vi "Command Editor Dialog.vi"(7 "Name(\"\" to use uuid)":string="Event CSM Tiny", 8 "Error in":errorcluster caption="Error in (no error)", 11 "Command":string="UI: Front Panel State >> Open -@ abc") -> (0 "Error out":errorcluster, 3 "Command out":string)   [LabVIEW 2017]
uses:
  _Polymophic/Build Message with Arguments(Auto Check).vi
  _Support/Common/Trim Single line Text.vi
  AdvanceAPI/CSM - Break Down Multiple States String.vi
  AdvanceAPI/CSM - Compact Multiple States.vi
  AdvanceAPI/CSM - Keywords.vi
  _Support/CSMQ/_CSMOFGV.vi
  _Support/Message/Parse State with Arguments String.vi
  Communicable State Machine.lvlib
  _csmHelper/API with lvcsm Support/CSM-Helper API with lvcsm Support.lvlib
panel:
  in  "State":string(combo)
  in  "Argument":string(combo)
  in  "symbol":string(combo)
  in  "Target":string(combo)
  in  "Comments":string
  in  "CSM VI Def":string(combo)
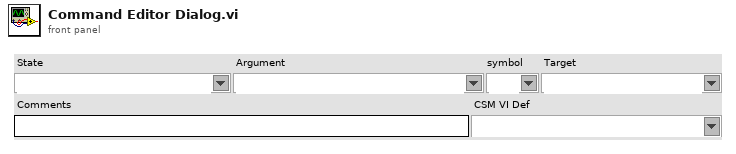
[diagram p1: front panel]
types:
  T1 = enum32{"Invalid", "Standard", "Closed", "Hidden", "Minimized", "Maximized"}
  T2 = enum32{"invalid app kind", "Development System", "Run Time System", "Student Edition", "Embedded LabVIEW", "Evaluation", "Custom"}
  T3 = typedef "Communicable State Machine.lvlib/_CSM_Response Source Message.ctl" = cluster{"‘State":string, "’Arguments":string, "’Error":errorcluster}
  T4 = cluster{"Current VI Reference":refnum<vi>, "Close Panel on Exit?":bool}
  T5 = cluster{"Core":cluster{"Current VI Reference":refnum<vi>, "Close Panel on Exit?":bool}, "Command":string}
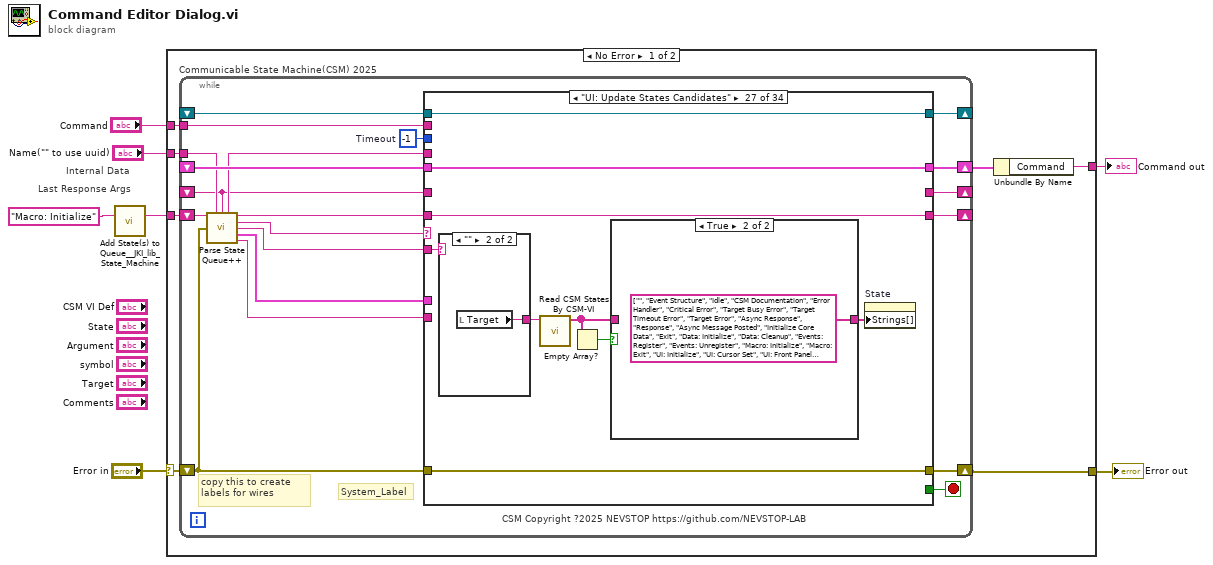
[diagram p0: block diagram]
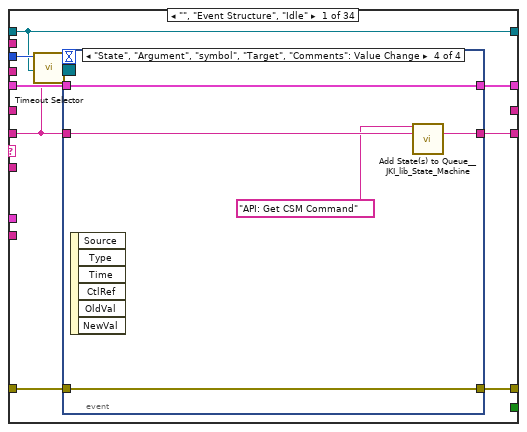
[diagram p2: hidden frame]
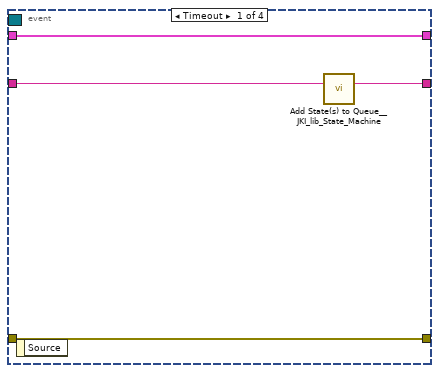
[diagram p3: hidden frame]
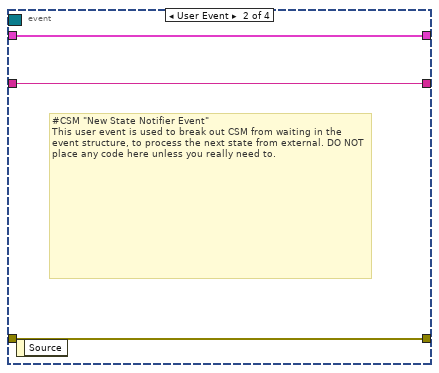
[diagram p4: hidden frame]
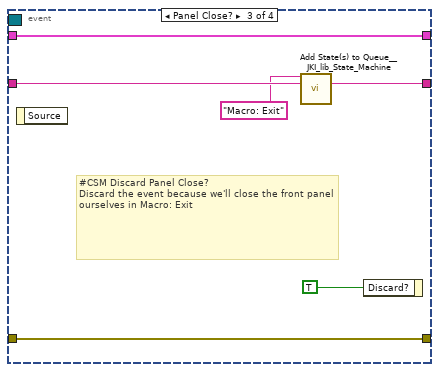
[diagram p5: hidden frame]
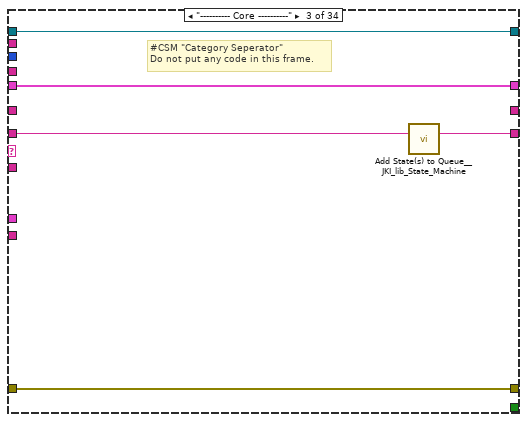
[diagram p7: hidden frame]
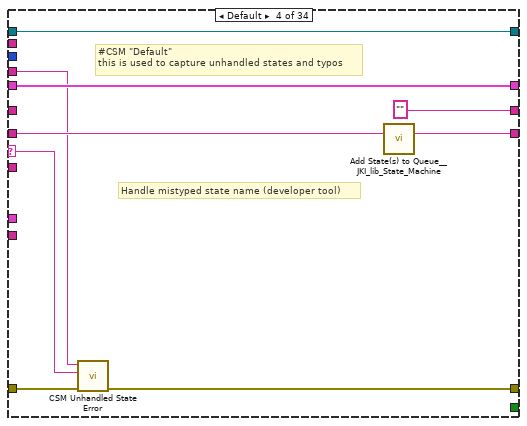
[diagram p8: hidden frame]
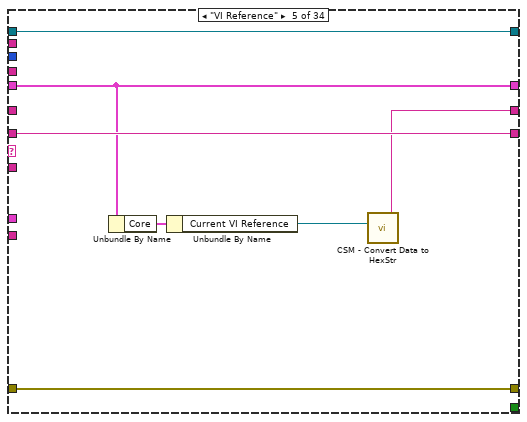
[diagram p9: hidden frame]
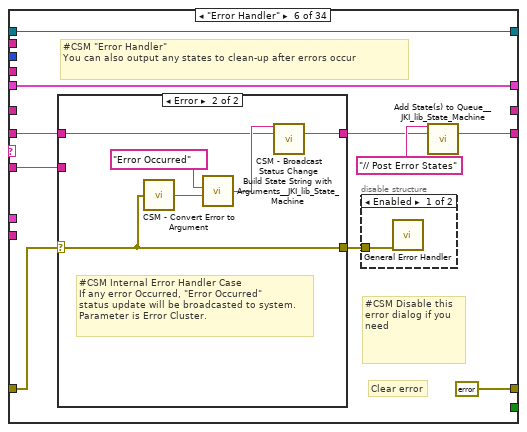
[diagram p10: hidden frame]
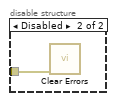
[diagram p11: hidden frame]
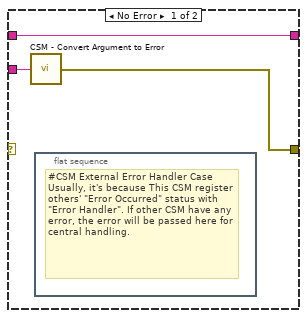
[diagram p12: hidden frame]
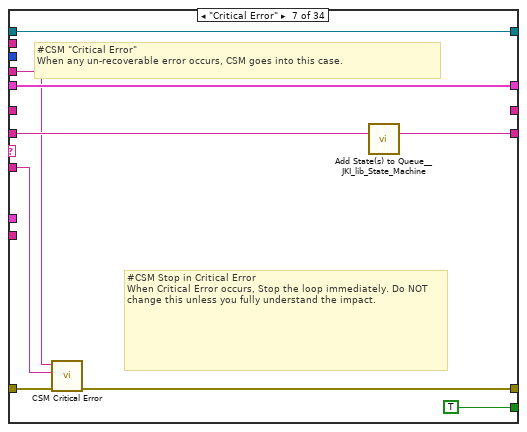
[diagram p13: hidden frame]
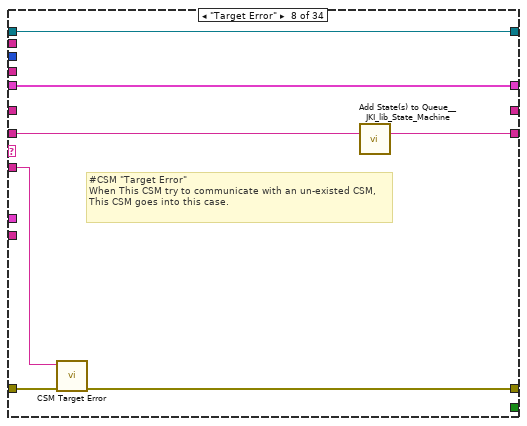
[diagram p14: hidden frame]
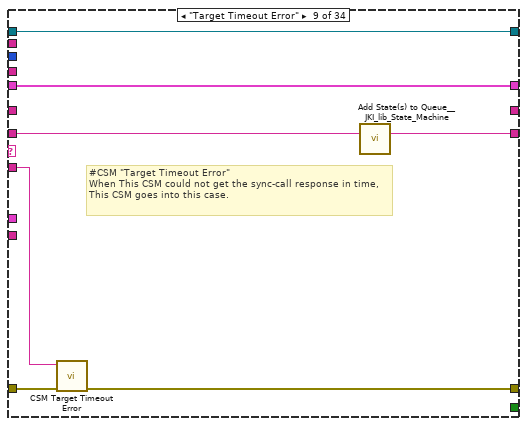
[diagram p15: hidden frame]
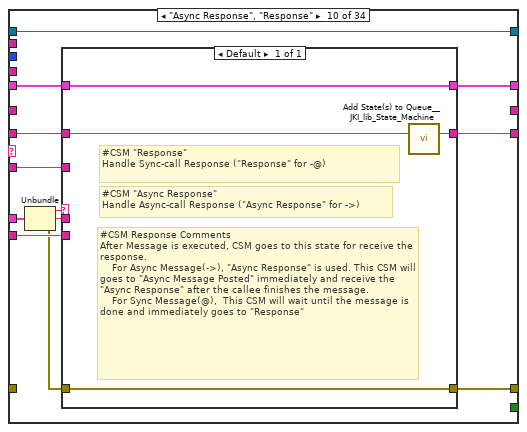
[diagram p16: hidden frame]
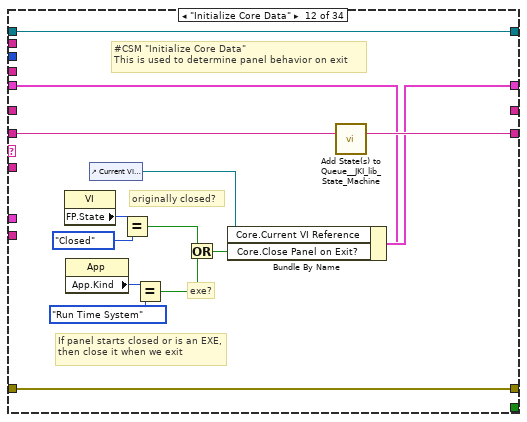
[diagram p18: hidden frame]
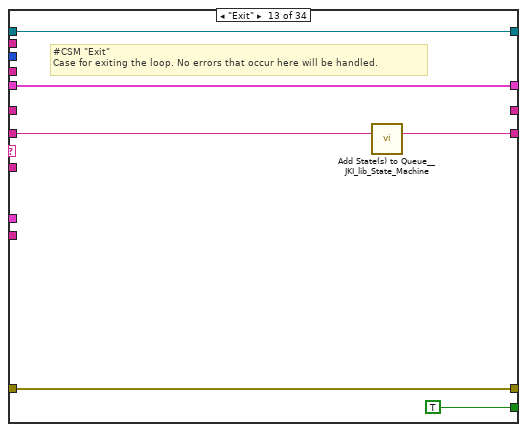
[diagram p19: hidden frame]
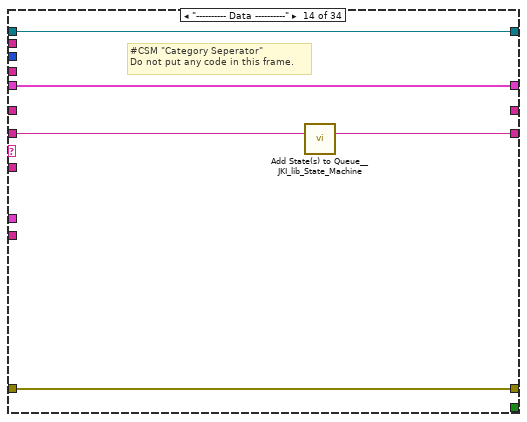
[diagram p20: hidden frame]
diagram:
  # "Last Response Args"
  # "Internal Data"
  n1 = call <vilib>:"Add State(s) to Queue__JKI_lib_State_Machine.vi"("State(s) in (\"\")"="Macro: Initialize" ("Init State(\"Macro: Initialize\")")) -> ("States Out"=w7:string)  [unwired: 14 in]
  n2 = case shown="No Error" "Error in" {
    selector: "Error in" -> [w11 w405]
    tunnel: w7 -> [w14 _]
    tunnel: "Name(\"\" to use uuid)" -> [w13 _]
    tunnel: [w12 w405] -> w4
    tunnel: [w9 w404] -> w2
    tunnel: "Command" -> [w8 w404]
    frame No Error {
      n3 = while "Communicable State Machine(CSM) 2025" {
        shift-right: [w29] -> w10
        shift-left: _ -> [w28]
        shift-right: [w32] -> w12
        shift-left: w11 -> [w26]
        shift-right: [w31] -> _
        shift-left: w14 -> [w33]
        tunnel: w13 -> [w22]
        shift-right: [w25] -> _
        shift-left: _ -> [w16]
        shift-right: [w24] -> _
        shift-left: _ -> [w23]
        tunnel: w8 -> [w15]
        stop <- w30 stop-if-true
        w27 = -1  # Timeout
        # "copy this to create labels for wires"
        # "System_Label"
        # "CSM Copyright ?2025 NEVSTOP https://github.com/NEVSTOP-LAB"
        n4 = call "Parse State Queue++.vi"("State Queue"=w33, "Name(\"\" to use uuid)"=w22, "Response Arguments"=w16, "Previous Error"=w26) -> ("Name Used"=w17:string, "Remaining States"=w34:string, "Current State"=w21:string, "Arguments"=w20:string, ">> Response Source Message >>"=w19:T3, ">> Source CSM >>"=w18:string)  [unwired: 6 in]
        n5 = case shown="\"UI: Update States Candidates\"" w21 {
          selector: w21 -> [_ _ _ w73 _ _ _ _ _ _ _ _ _ _ _ _ _ _ _ _ _ _ _ _ _ _ _ _ _ _ _ _ _ _]
          tunnel: w34 -> [w35 w64 w70 w78 w85 w91 w114 w120 w127 w136 w149 w164 w170 w175 w182 w189 w194 w201 w205 w211 w216 w230 w238 w254 w323 w328 w337 w347 w353 w365 w368 w371 w392 w403]
          tunnel: w20 -> [_ _ _ _ _ w90 w109 w119 w126 w135 _ _ _ _ _ _ _ _ _ _ _ _ w233 w248 _ _ w334 _ _ _ _ w373 _ _]
          tunnel: w28 -> [w42 w63 w67 w76 w84 w95 w115 w122 w129 w138 w148 w157 w168 w172 _ w184 w191 w200 w204 w208 w212 w218 w236 w250 w322 w327 w336 w344 w350 w362 w367 w377 w391 w400]
          tunnel: [w41 w65 w68 w71 w86 errorcluster {"status"=FALSE, "code"=0, "source"=""} ("error out") w110 w117 w124 w141 w150 w161 w167 w173 w179 w185 w192 w195 w203 w209 w214 w231 w234 w251 w324 w329 w338 w345 w351 w363 w369 w378 w393 w401] -> w32
          tunnel: w26 -> [w40 w65 w68 w79 w86 w92 w116 w118 w125 _ w150 w161 w167 w173 w179 w186 w192 _ w206 w209 w214 w231 w235 w252 w324 w329 w338 w345 w351 w363 w369 w378 w393 w401]
          tunnel: [w43 w64 w69 w77 w85 w87 w113 w123 w130 w137 w149 w163 w169 w174 w181 w188 w193 w201 w205 w210 w215 w230 w237 w253 w323 w328 w337 w346 w352 w364 w368 w372 w392 w402] -> w31
          tunnel: [_ _ _ _ _ _ TRUE _ _ _ _ _ TRUE _ _ _ _ _ _ _ _ _ _ _ _ _ _ _ _ _ _ _ _ _] -> w30
          tunnel: [w39 w63 w67 w76 w84 w95 w115 w122 w129 w139 w148 w162 w168 w172 w180 w184 w191 w200 w204 w208 w212 w218 w236 w250 w322 w327 w336 w344 w350 w362 w367 w375 w380 w400] -> w29
          tunnel: w27 -> [w38 _ _ _ _ _ _ _ _ _ _ _ _ _ _ _ _ _ _ _ _ _ _ _ _ _ _ _ _ _ _ _ _ _]
          tunnel: w18 -> [_ _ _ _ _ _ _ _ _ w133 _ _ _ _ _ _ _ _ _ _ _ _ _ _ _ _ _ _ _ _ _ _ _ _]
          tunnel: w19 -> [_ _ _ _ _ _ _ _ _ w140 _ _ _ _ _ _ _ _ _ _ _ _ _ _ _ _ _ _ _ _ _ _ _ _]
          tunnel: [_ _ _ "" w80 _ _ _ _ _ _ _ _ _ _ _ _ _ _ _ _ _ _ _ _ _ _ _ _ _ _ _ w386 _] -> w25
          tunnel: [w37 w62 w66 w74 w83 w94 w111 w121 w128 w142 w147 w151 w165 w171 w177 w183 w190 w199 w202 w207 w213 w229 w232 w247 w321 w326 w335 w343 w348 w355 w366 w376 w390 w399] -> w24
          tunnel: w23 -> [w37 w62 w66 w74 w83 w94 w111 w121 w128 w142 w147 w151 w165 w171 w177 w183 w190 _ w202 w207 w213 w229 w232 w247 w321 w326 w335 w343 w348 w355 w366 w376 w390 w399]
          tunnel: w17 -> [_ _ _ w72 _ _ w108 _ _ _ _ _ _ _ _ _ _ w198 _ _ _ _ _ _ _ _ _ _ _ _ _ _ _ _]
          tunnel: w16 -> [_ _ _ _ _ _ _ _ _ _ _ _ _ _ _ _ _ _ _ _ _ _ _ _ _ _ _ _ _ _ _ _ _ _]
          tunnel: w15 -> [_ _ _ _ _ _ _ _ _ _ _ _ _ _ w176 _ _ _ _ _ _ _ _ _ _ _ _ _ _ _ _ _ _ _]
          frame "", "Event Structure", "Idle" {
            n6 = call "Timeout Selector.vi"("Remaining States"=w35, "Timeout Expected"=w38) -> ("Timeout"=w36:i32)  [unwired: 5 in]
            n7 = event shown="[3] \"State\", \"Argument\", \"symbol\", \"Target\", \"Comments\": Value Change" {
              selector: w37 -> [_ _ _ _]
              dyn-events: _ -> [_ _ _ _]
              timeout: w36 -> [_ _ _ _]
              tunnel: w35 -> [w47 w49 w56 w58]
              tunnel: [w46 w49 w55 w59] -> w43
              tunnel: w42 -> [w44 w50 w53 w60]
              tunnel: [w45 w48 w54 w61] -> w41
              tunnel: w40 -> [w45 w48 w54 w61]
              tunnel: [w44 w50 w53 w60] -> w39
              event Timeout {
                n8 = event-data() -> ()  [unwired: 1 in, 1 out]
                n9 = call <vilib>:"Add State(s) to Queue__JKI_lib_State_Machine.vi"("State(s) in (\"\")"=w47) -> ("States Out"=w46:string)  [unwired: 14 in]
              }
              event User Event {
                # "#CSM \"New State Notifier Event\"\nThis user event is used to break out CSM from waiting in the event structure, to process the next state from external. DO NOT place any code here unless you really need to."
                n10 = event-data() -> ()  [unwired: 1 in, 1 out]
              }
              event Panel Close? {
                # "#CSM Discard Panel Close?\nDiscard the event because we'll close the front panel ourselves in Macro: Exit"
                n11 = event-data() -> ()  [unwired: 1 in, 1 out]
                n12 = call <vilib>:"Add State(s) to Queue__JKI_lib_State_Machine.vi"("State(s) in Front (\"\")"="Macro: Exit", "State(s) in (\"\")"=w56) -> ("States Out"=w55:string)  [unwired: 13 in]
                n13 = event-data("Discard?"=TRUE) -> ()  [unwired: 1 in, 1 out]
              }
              event "State", "Argument", "symbol", "Target", "Comments": Value Change {
                n14 = event-data() -> ()  [unwired: 1 in, 6 out]
                n15 = call <vilib>:"Add State(s) to Queue__JKI_lib_State_Machine.vi"("State(s) in Front (\"\")"="API: Get CSM Command" ("State(s) in Front (\"\")"), "State(s) in (\"\")"=w58) -> ("States Out"=w59:string)  [unwired: 13 in]
              }
            }
          }
          frame "CSM Documentation" {
            # "#CSM README FIRST\n\nCommunicable State Machine(CSM) is a LabVIEW application framework that builds upon JKI State Machine(JKISM). It follows the pattern of JKISM and extends the keywords to describe message communication between modules, including concepts such as Sync-Message, Async-Message, Subscription/Unsubscription of status - essential elements for creating reusable code modules. For more information, please visit the CSM wiki: https://nevstop-lab.github.io/CSM-Wiki/\n\nFor instructions on JKI State Machine, visit: http://jki.net/state-machine/\nFor information about CSM, visit: https://github.com/NEVSTOP-LAB"
            # "#CSM \"Documentation\"\nCase for holding CSM Documenation"
          }
          frame "---------- Core ----------" {
            # "#CSM \"Category Seperator\"\nDo not put any code in this frame."
            n16 = call <vilib>:"Add State(s) to Queue__JKI_lib_State_Machine.vi"("State(s) in (\"\")"=w70) -> ("States Out"=w69:string)  [unwired: 14 in]
          }
          frame Default {
            # "#CSM \"Default\"\nthis is used to capture unhandled states and typos"
            # "Handle mistyped state name (developer tool)"
            n17 = call "CSM Unhandled State Error.vi"("error in (no error)"=w79, "Current State"=w73, "CSM Name"=w72) -> ("error out"=w71:errorcluster)  [unwired: 8 in]
            n18 = call <vilib>:"Add State(s) to Queue__JKI_lib_State_Machine.vi"("State(s) in (\"\")"=w78) -> ("States Out"=w77:string)  [unwired: 14 in]
          }
          frame "VI Reference" {
            n19 = Unbundle By Name(w84) -> ("Core"=w82:T4)
            n20 = Unbundle By Name(w82) -> ("Current VI Reference"=w81:refnum<vi>)
            n21 = call "CSM - Convert Data to HexStr.vi"("Variant"=w81) -> ("HEX String (0-9,A-F)"=w80:string)  [unwired: 8 in]
          }
          frame "Error Handler" {
            # "#CSM Disable this error dialog if you need"
            # "#CSM \"Error Handler\"\nYou can also output any states to clean-up after errors occur"
            # "Clear error"
            n22 = case shown="Error" w92 {
              selector: w92 -> [_ w102]
              tunnel: [w101 w104] -> w88
              tunnel: w91 -> [w101 w103]
              tunnel: w90 -> [w100 _]
              tunnel: [w99 w102] -> w93
              frame No Error {
                n23 = call "CSM - Convert Argument to Error.vi"("Argument"=w100) -> ("error"=w99:errorcluster)  [unwired: 4 in]
                n24 = flat-sequence {
                  frame #0 {
                    # "#CSM External Error Handler Case\nUsually, it's because This CSM register others' \"Error Occurred\" status with \"Error Handler\". If other CSM have any error, the error will be passed here for central handling."
                  }
                }
              }
              frame Error {
                # "#CSM Internal Error Handler Case \nIf any error Occurred, \"Error Occurred\" \nstatus update will be broadcasted to system.\nParameter is Error Cluster."
                n25 = call "CSM - Convert Error to Argument.vi"("error"=w102) -> ("Argument"=w106:string)  [unwired: 4 in]
                n26 = call <vilib>:"Build State String with Arguments__JKI_lib_State_Machine.vi"("Arguments (\"\")"=w106, "State"="Error Occurred" ("Status with Arguments")) -> ("State with Arguments"=w105:string)  [unwired: 4 in]
                n27 = call "CSM - Broadcast Status Change.vi"("Status with Arguments"=w105, "State Queue"=w103) -> ("Remaining States"=w104:string)  [unwired: 13 in]
              }
            }
            n28 = disable-structure shown="Enabled" {
              disable-tunnel: w93 -> [w97 w98]
              frame Enabled {
                n29 = call <vilib>:"General Error Handler.vi"("error in (no error)"=w97) -> ()  [unwired: 10 in, 5 out]
              }
              frame Disabled {
                n30 = call <vilib>:"Clear Errors.vi"("error in (no error)"=w98) -> ()  [unwired: 5 in, 2 out]
              }
            }
            n31 = call <vilib>:"Add State(s) to Queue__JKI_lib_State_Machine.vi"("State(s) in Front (\"\")"="// Post Error States", "State(s) in (\"\")"=w88) -> ("States Out"=w87:string)  [unwired: 13 in]
          }
          frame "Critical Error" {
            # "#CSM Stop in Critical Error\nWhen Critical Error occurs, Stop the loop immediately. Do NOT change this unless you fully understand the impact."
            # "#CSM \"Critical Error\"\nWhen any un-recoverable error occurs, CSM goes into this case."
            n32 = call "CSM Critical Error.vi"("error in (no error)"=w116, "Arugments(as Reason)"=w109, "CSM Name"=w108) -> ("error out"=w110:errorcluster)  [unwired: 8 in]
            n33 = call <vilib>:"Add State(s) to Queue__JKI_lib_State_Machine.vi"("State(s) in (\"\")"=w114) -> ("States Out"=w113:string)  [unwired: 14 in]
          }
          frame "Target Error" {
            # "#CSM \"Target Error\"\nWhen This CSM try to communicate with an un-existed CSM, This CSM goes into this case."
            n34 = call "CSM Target Error.vi"("error in (no error)"=w118, "Arguments(as CSM Name)"=w119) -> ("error out"=w117:errorcluster)  [unwired: 9 in]
            n35 = call <vilib>:"Add State(s) to Queue__JKI_lib_State_Machine.vi"("State(s) in (\"\")"=w120) -> ("States Out"=w123:string)  [unwired: 14 in]
          }
          frame "Target Timeout Error" {
            # "#CSM \"Target Timeout Error\"\nWhen This CSM could not get the sync-call response in time, This CSM goes into this case."
            n36 = call "CSM Target Timeout Error.vi"("error in (no error)"=w125, "Arguments(as CSM Name)"=w126) -> ("error out"=w124:errorcluster)  [unwired: 9 in]
            n37 = call <vilib>:"Add State(s) to Queue__JKI_lib_State_Machine.vi"("State(s) in (\"\")"=w127) -> ("States Out"=w130:string)  [unwired: 14 in]
          }
          frame "Async Response", "Response" {
            n38 = Unbundle(w140) -> ("‘State"=w134:string, "’Arguments"=w132:string, "’Error"=w131:errorcluster)
            n39 = case shown="Default" w134 {
              tunnel: [w146] -> w141
              tunnel: w131 -> [w146]
              tunnel: [w145] -> w139
              tunnel: w138 -> [w145]
              tunnel: [w143] -> w137
              tunnel: w136 -> [w144]
              tunnel: w135 -> [_]
              tunnel: w133 -> [_]
              tunnel: w132 -> [_]
              frame Default {
                # "#CSM Response Comments\nAfter Message is executed, CSM goes to this state for receive the response.\n    For Async Message(->), \"Async Response\" is used. This CSM will goes to \"Async Message Posted\" immediately and receive the \"Async Response\" after the callee finishes the message.\n    For Sync Message(@),  This CSM will wait until the message is done and immediately goes to \"Response\""
                # "#CSM \"Async Response\"\nHandle Async-call Response (\"Async Response\" for ->)"
                # "#CSM \"Response\"\nHandle Sync-call Response (\"Response\" for -@)"
                n40 = call <vilib>:"Add State(s) to Queue__JKI_lib_State_Machine.vi"("State(s) in (\"\")"=w144) -> ("States Out"=w143:string)  [unwired: 14 in]
              }
            }
          }
          frame "Async Message Posted" {
            # "#CSM \"Async Message Posted\"\nAfter Async Message is posted (-> or ->| ), CSM goes to this state for post-action.\nYou can use Argument - State to tell which Async Message is called."
          }
          frame "Initialize Core Data" {
            # "#CSM \"Initialize Core Data\"\nThis is used to determine panel behavior on exit"
            # "originally closed?"
            # "exe?"
            # "If panel starts closed or is an EXE, then close it when we exit"
            n41 = property class="VI"() -> ("FP.State"=w154:T1)  [unwired: 2 in, 2 out]
            n42 = property class="App"() -> ("App.Kind"=w160:T2)  [unwired: 2 in, 2 out]
            n43 = control-ref of="Current VI Reference"() -> (w155:refnum<vi>)
            n44 = Equal?(x=w154, y=T1."Closed" ("Front Panel Window:State")) -> (x = y?=w152:bool)
            n45 = Equal?(x=w160, y=T2."Run Time System" ("Application:Kind")) -> (x = y?=w158:bool)
            n46 = Or(x=w152, y=w158) -> (x .or. y?=w156:bool)
            n47 = Bundle By Name(cluster=w157, "Core.Current VI Reference"=w155, "Core.Close Panel on Exit?"=w156) -> (w162:T5)
            n48 = call <vilib>:"Add State(s) to Queue__JKI_lib_State_Machine.vi"("State(s) in (\"\")"=w164) -> ("States Out"=w163:string)  [unwired: 14 in]
          }
          frame "Exit" {
            # "#CSM \"Exit\"\nCase for exiting the loop. No errors that occur here will be handled."
            n49 = call <vilib>:"Add State(s) to Queue__JKI_lib_State_Machine.vi"("State(s) in (\"\")"=w170) -> ("States Out"=w169:string)  [unwired: 14 in]
          }
          frame "---------- Data ----------" {
            # "#CSM \"Category Seperator\"\nDo not put any code in this frame."
            n50 = call <vilib>:"Add State(s) to Queue__JKI_lib_State_Machine.vi"("State(s) in (\"\")"=w175) -> ("States Out"=w174:string)  [unwired: 14 in]
          }
          frame "Data: Initialize" {
            w178 = T4 {"Current VI Reference"=refnum, "Close Panel on Exit?"=FALSE}  # Core
            n51 = Bundle("Core"=w178, "Command"=w176) -> (w180:T5)  [unwired: 1 in]
            n52 = call <vilib>:"Add State(s) to Queue__JKI_lib_State_Machine.vi"("State(s) in (\"\")"=w182) -> ("States Out"=w181:string)  [unwired: 14 in]
          }
          frame "Data: Cleanup" {
            # "Cleanup any data and references, here.\n(this is called automatically, by the Macro: Exit)"
            n53 = Unbundle By Name(w184) -> ("Core.Current VI Reference"=w187:refnum<vi>)
            n54 = Close Reference(reference=w187, error in (no error)=w186) -> (error out=w185:errorcluster)
            n55 = call <vilib>:"Add State(s) to Queue__JKI_lib_State_Machine.vi"("State(s) in (\"\")"=w189) -> ("States Out"=w188:string)  [unwired: 14 in]
          }
          frame "---------- Events ----------" {
            # "#CSM \"Category Seperator\"\nDo not put any code in this frame."
            n56 = call <vilib>:"Add State(s) to Queue__JKI_lib_State_Machine.vi"("State(s) in (\"\")"=w194) -> ("States Out"=w193:string)  [unwired: 14 in]
          }
          frame "Events: Register" {
            # "#CSM \"Events: Register\"\nRegister user event. New Message Event is registered to break CSM waiting in event structure by default."
            # "#CSM Register New Message Event\nRegister message event to break Waiting in Event structure."
            n57 = call "CSM - Get New State Notifier Event.vi"("Name(\"\" to use uuid) in"=w198) -> ("Error out"=w196:errorcluster, "New State Notifier Event"=w197:refnum<user-event>)  [unwired: 9 in]
            n58 = register-events(error in=w196, w197) -> (reference out=w199:refnum<event-registration>, error out=w195:errorcluster)  [unwired: 1 in]
          }
          frame "Events: Unregister" {
            # "#CSM \"Events: Unregister\"\nUnregister user event."
            n59 = Unregister For Events(event registration refnum=w202, error in=w206) -> (error out=w203:errorcluster)
          }
          frame "---------- UI ----------" {
            # "#CSM \"Category Seperator\"\nDo not put any code in this frame."
            n60 = call <vilib>:"Add State(s) to Queue__JKI_lib_State_Machine.vi"("State(s) in (\"\")"=w211) -> ("States Out"=w210:string)  [unwired: 14 in]
          }
          frame "UI: Initialize" {
            # "#CSM \"UI: Initialize\"\nInitialize the User Interface, here.\n(this is called automatically, by the Macro: Init)"
            n61 = call <vilib>:"Add State(s) to Queue__JKI_lib_State_Machine.vi"("State(s) in (\"\")"=w216) -> ("States Out"=w215:string)  [unwired: 14 in]
          }
          frame "UI: Refresh Inputs" {
            n62 = Unbundle By Name(w218) -> ("Command"=w217:string)
            n63 = call "Remove Comments from Line.vi"("single-line text"=w217) -> ("single-line text without comments"=w223:string)  [unwired: 2 in]
            n64 = call "Splite Single-line Message.vi"("single-line text"=w223) -> ("operator"=w228:string, "state"=w227:string, "args"=w226:string, "source/target"=w225:string)  [unwired: 6 in]
            n65 = String Length(string=w223) -> (length=w224:i32)
            n66 = String Subset(string=w217, offset (0)=w224) -> (substring=w221:string)  [unwired: 1 in]
            n67 = call "Trim Both Whitespace.vi"("string"=w221) -> ("trimmed string"=w220:string)  [unwired: 1 in]
            n68 = Match Pattern(string=w220, regular expression="^[/][/]+") -> (after substring=w222:string)  [unwired: 1 in, 3 out]
            n69 = local write "State"(w227) -> ()
            n70 = local write "Argument"(w226) -> ()
            n71 = local write "symbol"(w228) -> ()
            n72 = local write "Comments"(w222) -> ()
            n73 = local write "Target"(w225) -> ()
          }
          frame "UI: Cursor Set" {
            # "#CSM \"UI: Cursor Set\"\nSet and Unset Cursor Busy.\n(Usage: \"UI: Cursor Set >> Busy|Idle\")"
            # "Argument"
            n74 = disable-structure shown="Default" {
              disable-tunnel: w235 -> [w241 w246]
              disable-tunnel: [w240 w246] -> w234
              disable-tunnel: w233 -> [w239 _]
              frame condition #0 (active) {
                n75 = case shown="\"Idle\", Default" w239 {
                  tunnel: w241 -> [w243 w245]
                  tunnel: [w242 w244] -> w240
                  frame "Idle", Default {
                    n76 = call <vilib>:"Unset Busy.vi"("error in (no error)"=w243) -> ("error out"=w242:errorcluster)  [unwired: 10 in]
                  }
                  frame "Busy" {
                    n77 = call <vilib>:"Set Busy.vi"("error in (no error)"=w245) -> ("error out"=w244:errorcluster)  [unwired: 9 in, 1 out]
                  }
                }
              }
              frame condition #1 {
              }
            }
            n78 = call <vilib>:"Add State(s) to Queue__JKI_lib_State_Machine.vi"("State(s) in (\"\")"=w238) -> ("States Out"=w237:string)  [unwired: 14 in]
          }
          frame "UI: Front Panel State" {
            # "#CSM \"UI: Front Panel State\"\nSet Front Panel Open or Closed\n(Usage: \"UI: Front Panel State >> Open|Close\")"
            # "Argument"
            n79 = Unbundle By Name(w250) -> ("Core.Current VI Reference"=w249:refnum<vi>)
            n80 = call <vilib>:"Add State(s) to Queue__JKI_lib_State_Machine.vi"("State(s) in (\"\")"=w254) -> ("States Out"=w253:string)  [unwired: 14 in]
            n81 = case shown="\"Close\", \"Closed\"" w248 {
              tunnel: w252 -> [w260 w275 w286 w299 w312]
              tunnel: [w262 w276 w288 w301 w314] -> w251
              tunnel: w249 -> [w261 w273 w287 w300 w313]
              frame "Open", "Standard", Default {
                w255 = T1."Standard" ("State")
                n82 = property class="VI"(reference=w261, error in=w260) -> (reference out=w258:refnum<vi>, error out=w259:errorcluster, "FP.State"=w257:T1)
                n83 = Not Equal?(x=w257, y=w255) -> (x != y?=w256:bool)
                n84 = case shown="True" w256 {
                  tunnel: [w266 w268] -> w262
                  tunnel: w259 -> [w265 w268]
                  tunnel: w258 -> [w264 _]
                  tunnel: w255 -> [w263 _]
                  frame True {
                    n85 = invoke class="VI" method="FP.Open"(reference=w264, error in=w265, "Activate"=TRUE, "State"=w263) -> (error out=w266:errorcluster)  [unwired: 1 in, 4 out]
                  }
                  frame False {
                  }
                }
              }
              frame "Close", "Closed" {
                n86 = property class="VI"(reference=w273, error in=w275) -> (reference out=w272:refnum<vi>, error out=w274:errorcluster, "FP.State"=w270:T1)
                n87 = Not Equal?(x=w270, y=T1."Closed" ("Front Panel Window:State")) -> (x != y?=w269:bool)
                n88 = case shown="False" w269 {
                  tunnel: [w277 w280] -> w276
                  tunnel: w274 -> [w277 w279]
                  tunnel: w272 -> [_ w278]
                  frame False {
                  }
                  frame True {
                    n89 = invoke class="VI" method="FP.Close"(reference=w278, error in=w279) -> (error out=w280:errorcluster)  [unwired: 1 in, 2 out]
                  }
                }
              }
              frame "Hidden", "Hide" {
                w281 = T1."Hidden" ("State")
                n90 = property class="VI"(reference=w287, error in=w286) -> (reference out=w284:refnum<vi>, error out=w285:errorcluster, "FP.State"=w283:T1)
                n91 = Not Equal?(x=w283, y=w281) -> (x != y?=w282:bool)
                n92 = case shown="True" w282 {
                  tunnel: [w292 w293] -> w288
                  tunnel: w285 -> [w291 w293]
                  tunnel: w284 -> [w290 _]
                  tunnel: w281 -> [w289 _]
                  frame True {
                    n93 = invoke class="VI" method="FP.Open"(reference=w290, error in=w291, "State"=w289) -> (error out=w292:errorcluster)  [unwired: 2 in, 4 out]
                  }
                  frame False {
                  }
                }
              }
              frame "Minimize", "Minimized" {
                w294 = T1."Minimized" ("State")
                n94 = property class="VI"(reference=w300, error in=w299) -> (reference out=w297:refnum<vi>, error out=w298:errorcluster, "FP.State"=w296:T1)
                n95 = Not Equal?(x=w296, y=w294) -> (x != y?=w295:bool)
                n96 = case shown="True" w295 {
                  tunnel: [w305 w306] -> w301
                  tunnel: w298 -> [w304 w306]
                  tunnel: w297 -> [w303 _]
                  tunnel: w294 -> [w302 _]
                  frame True {
                    n97 = invoke class="VI" method="FP.Open"(reference=w303, error in=w304, "State"=w302) -> (error out=w305:errorcluster)  [unwired: 2 in, 4 out]
                  }
                  frame False {
                  }
                }
              }
              frame "Maximize", "Maximized" {
                w307 = T1."Maximized" ("State")
                n98 = property class="VI"(reference=w313, error in=w312) -> (reference out=w310:refnum<vi>, error out=w311:errorcluster, "FP.State"=w309:T1)
                n99 = Not Equal?(x=w309, y=w307) -> (x != y?=w308:bool)
                n100 = case shown="True" w308 {
                  tunnel: [w318 w319] -> w314
                  tunnel: w311 -> [w317 w319]
                  tunnel: w310 -> [w316 _]
                  tunnel: w307 -> [w315 _]
                  frame True {
                    n101 = invoke class="VI" method="FP.Open"(reference=w316, error in=w317, "State"=w315) -> (error out=w318:errorcluster)  [unwired: 2 in, 4 out]
                  }
                  frame False {
                  }
                }
              }
            }
          }
          frame "UI: Update CSM Candidates" {
            n102 = call "Read CSMs.vi"() -> ("Array"=w320:string[])  [unwired: 10 in, 1 out]
            n103 = property on="Target" class="CmbBox"("Strings[]"=w320) -> ()  [unwired: 2 in, 2 out]
          }
          frame "UI: Update CSM-VI Candidates" {
            n104 = call "Read CSM-VIs.vi"() -> ("Array"=w325:string[])  [unwired: 10 in, 1 out]
            n105 = property on="CSM-VI" class="CmbBox"("Strings[]"=w325) -> ()  [unwired: 2 in, 2 out]
          }
          frame "UI: Update States Candidates" {
            n106 = case shown="\"\"" w334 {
              selector: w334 -> [w341 _]
              tunnel: [w341 w342] -> w333
              frame Default {
              }
              frame "" {
                n107 = local read "Target"() -> (w342:string)
              }
            }
            n108 = call "Read CSM States By CSM-VI.vi"("CSM VI"=w333) -> ("Array"=w331:string[])  [unwired: 9 in, 1 out]
            n109 = Empty Array?(array=w331) -> (empty?=w332:bool)
            n110 = case shown="True" w332 {
              tunnel: w331 -> [w339 _]
              tunnel: [w339 string[] ["", "Event Structure", "Idle", "CSM Documentation", "Error Handler", "Critical Error", "Target Busy Error", "Target Timeout Error", "Target Error", "Async Response", "Response", "Async Message Posted", "Initialize Core Data", "Exit", "Data: Initialize", "Data: Cleanup", "Events: Register", "Events: Unregister", "Macro: Initialize", "Macro: Exit", "UI: Initialize", "UI: Cursor Set", "UI: Front Panel State", "Data: Get Configuration", "Data: Get Internal Data", "Data: Set Configuration", "Data: Update Indicators", "VI Reference"] ("items to filter")] -> w330
              frame False {
              }
              frame True {
              }
            }
            n111 = property on="State" class="CmbBox"("Strings[]"=w330) -> ()  [unwired: 2 in, 2 out]
          }
          frame "---------- Macro ----------" {
            # "#CSM \"Category Seperator\"\nDo not put any code in this frame."
            n112 = call <vilib>:"Add State(s) to Queue__JKI_lib_State_Machine.vi"("State(s) in (\"\")"=w347) -> ("States Out"=w346:string)  [unwired: 14 in]
          }
          frame "Macro: Initialize" {
            w349 = "Data: Initialize\nInitialize Core Data\nEvents: Register\nUI: Initialize\n//UI: Front Panel State >> Open\nUI: Refresh Inputs\nUI: Update CSM Candidates\nUI: Update CSM-VI Candidates\nUI: Update States Candidates"  # Data: Initialize Initialize Core Data Events: Register UI: Initialize //UI: Front Panel State >> Open UI: Refresh Inputs UI: Update CSM Candidates UI: Update CSM-VI Candidates UI: Update States Candidates
            # "#CSM \"Macro: Initialize\"\nInitialization Macro (This is called once, when the VI starts)"
            n113 = call <vilib>:"Add State(s) to Queue__JKI_lib_State_Machine.vi"("State(s) in Front (\"\")"=w349, "State(s) in (\"\")"=w353) -> ("States Out"=w352:string)  [unwired: 13 in]
          }
          frame "Macro: Exit" {
            # "#CSM \"Macro: Exit\"\nExit Macro (This is called once, when the VI exits)"
            n114 = Unbundle By Name(w362) -> ("Core.Close Panel on Exit?"=w361:bool)
            n115 = Select(t="UI: Front Panel State >> Close", s=w361, f="") -> (s? t:f=w358:string)
            n116 = call <vilib>:"Add State(s) to Queue__JKI_lib_State_Machine.vi"("State(s) in Front (\"\")"="//Exit Sub-Modules ", "State(s) in (\"\")"=w358, "State(s) at Back (\"\")"="Data: Cleanup\nEvents: Unregister\nExit") -> ("States Out"=w356:string)  [unwired: 12 in]
            n117 = call <vilib>:"Add State(s) to Queue__JKI_lib_State_Machine.vi"("State(s) in Front (\"\")"=w356, "State(s) in (\"\")"=w365) -> ("States Out"=w364:string)  [unwired: 13 in]
          }
          frame "---------- API ----------" {
            # "#CSM \"Category Seperator\"\nDo not put any code in this frame."
          }
          frame "API: Set Command" {
            # "#CSM API Example\nCopy/Rename this case for your own API"
            n118 = call "CSM - Revert Arguments-Safe String.vi"("Safe Argurment String"=w373) -> ("Origin Argurment String"=w374:string)  [unwired: 8 in]
            n119 = Bundle By Name(cluster=w377, "Command"=w374) -> (w375:T5)
            n120 = call <vilib>:"Add State(s) to Queue__JKI_lib_State_Machine.vi"("State(s) in (\"\")"=w371, "State(s) at Back (\"\")"="UI: Refresh Inputs" ("State(s) in Front (\"\")")) -> ("States Out"=w372:string)  [unwired: 13 in]
          }
          frame "API: Get CSM Command" {
            # "#CSM API Example\nCopy/Rename this case for your own API"
            n121 = local read "State"() -> (w383:string)
            n122 = local read "symbol"() -> (w384:string)
            n123 = local read "Comments"() -> (w388:string)
            n124 = local read "Argument"() -> (w385:string)
            n125 = local read "Target"() -> (w381:string)
            n126 = Concatenate Strings(w383, w384, w381) -> (w382:string)
            n127 = call-poly "Build Message with Arguments++.vi"("State with Arguments"=w382, "Arguments (\"\")"=w385, "Target Module (\"\")"=w381) -> ("CSM Message String"=w389:string)  [unwired: 12 in]
            n128 = case shown="\"\"" w388 {
              selector: w388 -> [_ w397]
              tunnel: w389 -> [w394 w398]
              tunnel: "  //" ("string") -> [_ w396]
              tunnel: [w394 w395] -> w379
              frame "" {
              }
              frame Default {
                n129 = Concatenate Strings(w398, w396, w397) -> (w395:string)
              }
            }
            n130 = Bundle By Name(cluster=w391, "Command"=w379) -> (w380:T5)
            n131 = call "CSM - Make String Arguments Safe.vi"("Argurment String"=w379) -> ("Safe Argurment String"=w386:string)  [unwired: 8 in]
          }
          frame "---------- Action ----------" {
            # "#CSM \"Category Seperator\"\nDo not put any code in this frame."
            n132 = call <vilib>:"Add State(s) to Queue__JKI_lib_State_Machine.vi"("State(s) in (\"\")"=w403) -> ("States Out"=w402:string)  [unwired: 14 in]
          }
        }
      }
      n133 = Unbundle By Name(w10) -> ("Command"=w9:string)
    }
    frame Error {
    }
  }
  "Error out" <- w4
  "Command out" <- w2
